vi "Set User and Repository.vi"(8 "error in (no error)":errorcluster, 9 "Repository":string, 10 "User":string, 11 "SelfUpdate in":refnum<class "SelfUpdate.lvclass">) -> (0 "error out":errorcluster, 3 "SelfUpdate out":refnum<class "SelfUpdate.lvclass">)   [LabVIEW 2013, in "SelfUpdate.lvclass"]
uses:
  SelfUpdate.lvclass
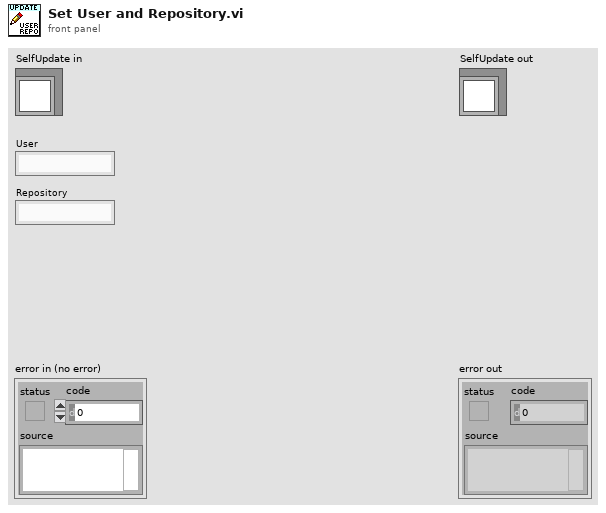
[diagram p1: front panel]
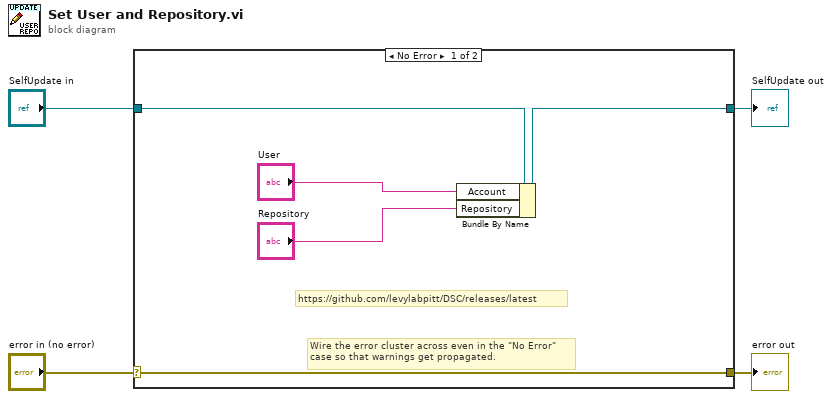
[diagram p0: block diagram]
diagram:
  n1 = case shown="No Error" "error in (no error)" {
    selector: "error in (no error)" -> [w9 w11]
    tunnel: [w9 w11] -> w3
    tunnel: [w7 w10] -> w1
    tunnel: "SelfUpdate in" -> [w8 w10]
    frame No Error {
      # "https://github.com/levylabpitt/DSC/releases/latest"
      # "Wire the error cluster across even in the \"No Error\"\ncase so that warnings get propagated."
      n2 = Bundle By Name(cluster=w8, "Account"="User", "Repository"="Repository") -> (w7:refnum<class "SelfUpdate.lvclass">)
    }
    frame Error {
    }
  }
  "error out" <- w3
  "SelfUpdate out" <- w1
